vi "PlaySound.vi"(8 "error in (no error)":errorcluster, 9 "Volume":dbl(slide)=50.0 scale=0.0..100.0, 10 "Duration (s)":dbl, 11 "Frequency":dbl=500.0) -> (0 "error out":errorcluster)   [LabVIEW 2022 SP3]
uses:
  <vilib>/sound2/lvsound2.llb/Sampling Mode.ctl
  <vilib>/sound2/lvsound2.llb/Sound Data Format.ctl
  <vilib>/sound2/lvsound2.llb/Sound Output Set Volume (Single).vi
  <vilib>/sound2/lvsound2.llb/Sound Output Write (DBL Single).vi
panel:
  in  "Stop":bool
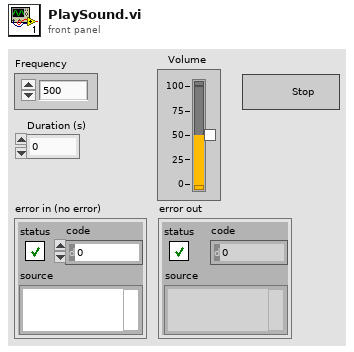
[diagram p1: front panel]
types:
  T1 = typedef "Sound Data Format.ctl" = cluster{"sample rate (S/s)":dbl, "number of channels":i32, "bits per sample":i32}
  T2 = typedef "Sampling Mode.ctl" = i32
  T3 = typedef "Sound Output Task ID.ctl" = u32
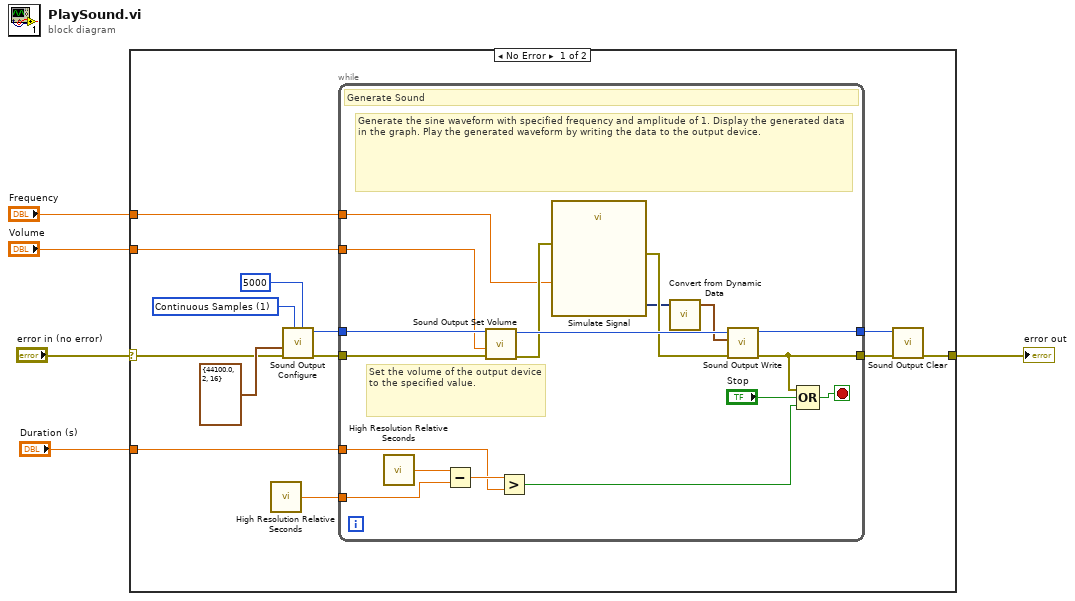
[diagram p0: block diagram]
diagram:
  n1 = case shown="No Error" "error in (no error)" {
    selector: "error in (no error)" -> [w6 w37]
    tunnel: "Volume" -> [w13 _]
    tunnel: "Frequency" -> [w12 _]
    tunnel: [w9 w37] -> w3
    tunnel: "Duration (s)" -> [w7 _]
    frame No Error {
      w17 = T2 1 items=["Finite Samples", "Continuous Samples"] ("sample mode")
      n2 = call <vilib>:"High Resolution Relative Seconds.vi"() -> ("relative seconds"=w8:dbl)
      n3 = call <vilib>:"Sound Output Configure.vi"("number of samples/ch"=5000, "sample mode"=w17, "error in (no error)"=w6, "sound format"=T1 {"sample rate (S/s)"=44100.0, "number of channels"=2, "bits per sample"=16}) -> ("error out"=w14:errorcluster, "task ID"=w15:T3)  [unwired: 6 in]
      n4 = while {
        tunnel: w15 -> [w31]
        tunnel: [w36] -> w10
        tunnel: w14 -> [w33]
        tunnel: [w30] -> w11
        tunnel: w13 -> [w25]
        tunnel: w12 -> [w24]
        tunnel: w8 -> [w22]
        tunnel: w7 -> [w20]
        stop <- w34 stop-if-true
        # "Set the volume of the output device to the specified value."
        # "Generate the sine waveform with specified frequency and amplitude of 1. Display the generated data in the graph. Play the generated waveform by writing the data to the output device."
        # "Generate Sound"
        n5 = call <vilib>:"High Resolution Relative Seconds.vi"() -> ("relative seconds"=w23:dbl)
        n6 = Subtract(x=w23, y=w22) -> (x-y=w21:dbl)
        n7 = call-poly <vilib>:"Sound Output Set Volume.vi"("error in (no error)"=w33, "volume"=w25, "task ID"=w31) -> ("error out"=w28:errorcluster, "task ID out"=w32:T3)  [unwired: 7 in]
        n8 = Greater?(x=w21, y=w20) -> (0:w19:bool)
        n9 = call "Simulate Signal"("Frequency"=w24, "error in (no error)"=w28) -> ("Sine"=w26:dynamicdata, "error out"=w27:errorcluster)  [unwired: 12 in]
        n10 = call "Convert from Dynamic Data"("Dynamic Data Type"=w26) -> ("Waveform"=w29:waveform(dbl))  [unwired: 3 in]
        n11 = call-poly <vilib>:"Sound Output Write.vi"("error in (no error)"=w27, "data"=w29, "task ID"=w32) -> ("error out"=w30:errorcluster, "task ID out"=w36:T3)  [unwired: 7 in]
        n12 = Compound Arithmetic op=OR(w30, "Stop", w19) -> (w34:bool)
      }
      n13 = call <vilib>:"Sound Output Clear.vi"("error in (no error)"=w11, "task ID"=w10) -> ("error out"=w9:errorcluster)  [unwired: 9 in]
    }
    frame Error {
    }
  }
  "error out" <- w3
